vi "NoteOnNoteOff.vi"() -> ()   [LabVIEW 2015]
panel:
  in  "which cap touch sensor":i32
  in  "play note (0/1)":i32
  out "output string: play":string
  out "output string: stop playing":string
  out "index of note, initial":i32[](array[numeric])
  out "index of note":i32[](array[numeric])
  out "10-element note values":i32[](array[numeric])
  out "Interate through 36 inputs":i32
  out "10-element note values, initial":i32[](array[numeric])
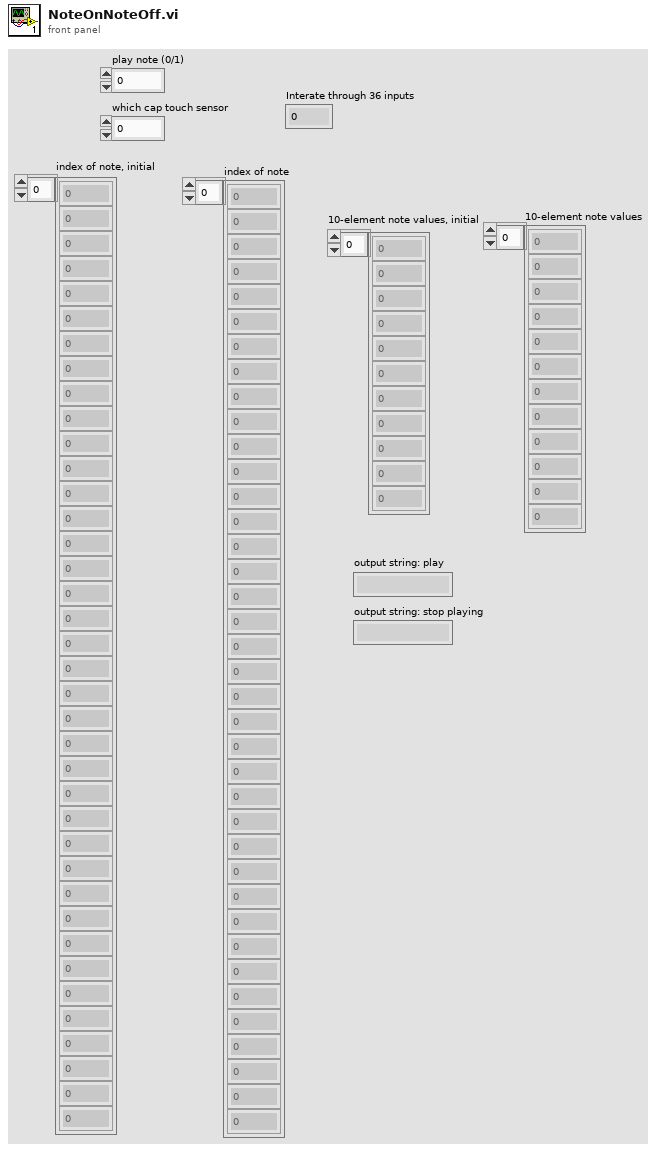
[diagram p1: front panel]
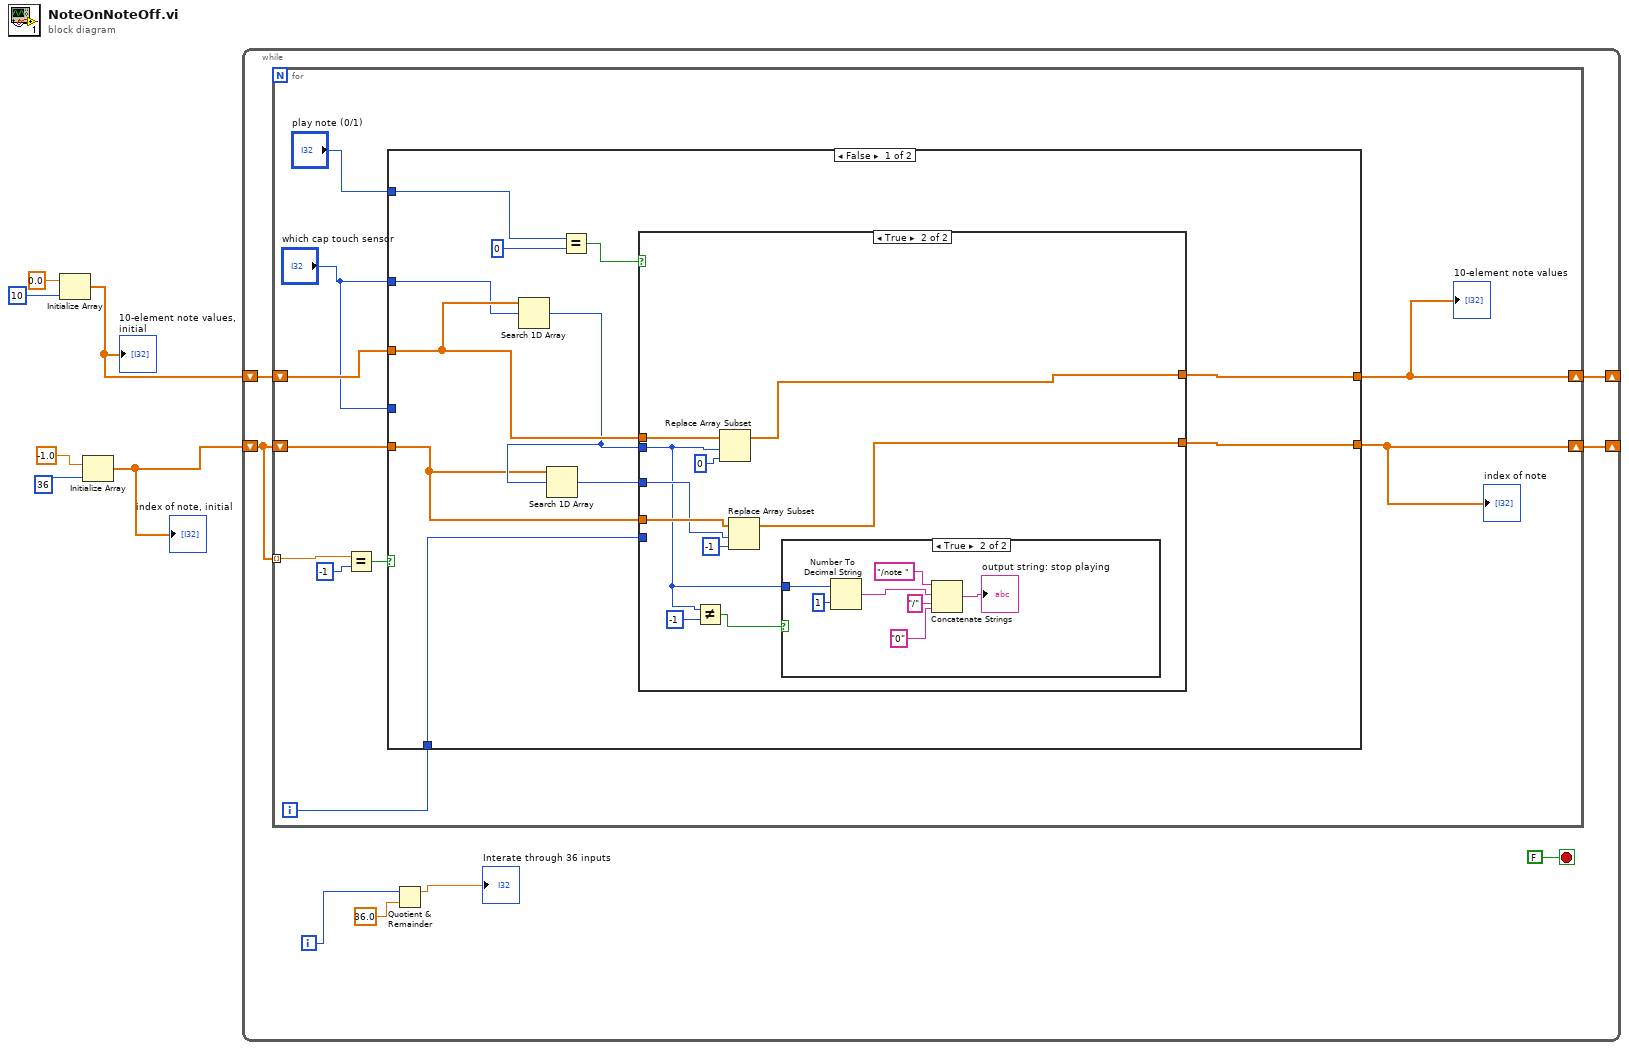
[diagram p0: block diagram]
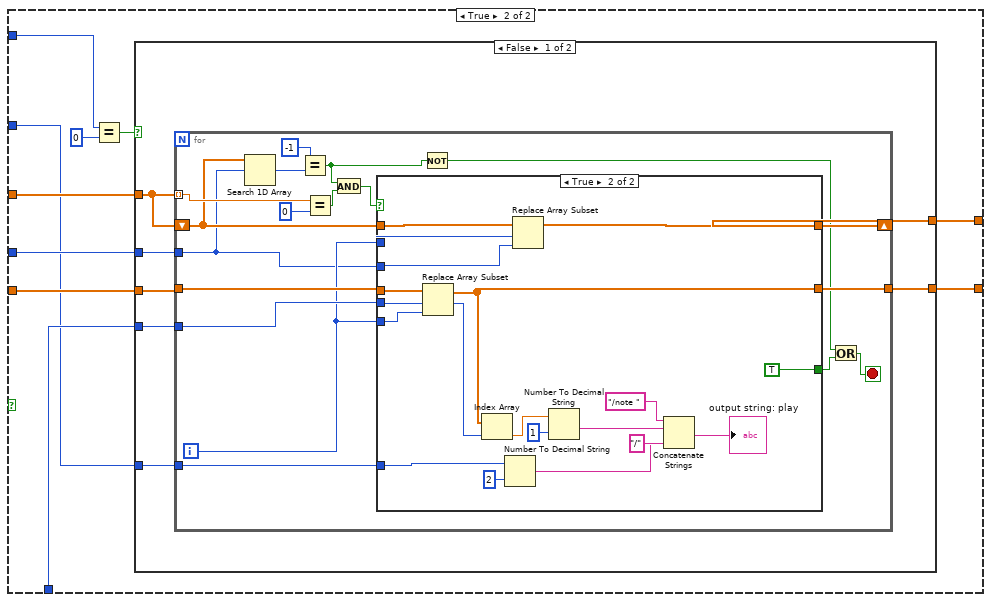
[diagram p4: hidden frame]
diagram:
  n1 = Initialize Array(0.0 ("element"), 10 ("dimension size")) -> (w1:dbl[])
  "10-element note values, initial" <- w1
  n2 = Initialize Array(-1.0 ("element"), 36 ("dimension size")) -> (w4:dbl[])
  "index of note, initial" <- w4
  n3 = while {
    shift-right: [w12] -> _
    shift-left: w1 -> [w14]
    shift-right: [w13] -> _
    shift-left: w4 -> [w10]
    i -> [w8]
    stop <- FALSE stop-if-true
    n4 = for {
      tunnel: w10 -> [w21] mode=indexing
      shift-right: [w18] -> w12
      shift-left: w14 -> [w24]
      shift-right: [w19] -> w13
      shift-left: w10 -> [w23]
      i -> [w15]
      n5 = Equal?(x=w21, y=-1) -> (x = y?=w20:bool)
      n6 = case shown="False" w20 {
        tunnel: "which cap touch sensor" -> [_ w64]
        tunnel: w24 -> [w29 w63]
        tunnel: w23 -> [w26 w62]
        tunnel: w15 -> [w34 w61]
        tunnel: "which cap touch sensor" -> [w28 w56]
        tunnel: [w32 w58] -> w18
        tunnel: [w31 w57] -> w19
        tunnel: "play note (0/1)" -> [w30 w55]
        frame False {
          n7 = Search 1D Array(1D array=w29, element=w28) -> (index of element=w27:i32)  [unwired: 1 in]
          n8 = Search 1D Array(1D array=w26, element=w27) -> (index of element=w25:i32)  [unwired: 1 in]
          n9 = Equal?(x=w30, y=0) -> (x = y?=w33:bool)
          n10 = case shown="True" w33 {
            tunnel: w29 -> [w37 w47]
            tunnel: w27 -> [_ w38]
            tunnel: w34 -> [_ _]
            tunnel: w26 -> [w36 w42]
            tunnel: [w37 w44] -> w32
            tunnel: [w36 w43] -> w31
            tunnel: w25 -> [_ w39]
            frame False {
            }
            frame True {
              n11 = Not Equal?(x=w38, y=-1) -> (x != y?=w40:bool)
              n12 = Replace Array Subset(array=w47, new element=0 ("new element/subarray"), index=w38) -> (w44:dbl[])
              n13 = Replace Array Subset(array=w42, new element=-1 ("new element/subarray"), index=w39) -> (w43:dbl[])
              n14 = case shown="True" w40 {
                tunnel: w38 -> [_ w48]
                frame False {
                }
                frame True {
                  n15 = Number To Decimal String(number=w48, width (-)=i16 1) -> (decimal integer string=w52:string)
                  n16 = Concatenate Strings("/note " ("string"), w52, "/" ("string"), "0" ("string")) -> (→"output string: stop playing":string)
                }
              }
            }
          }
        }
        frame True {
          n17 = Equal?(x=w55, y=0) -> (x = y?=w59:bool)
          n18 = case shown="False" w59 {
            tunnel: w64 -> [w71 _]
            tunnel: w63 -> [w70 w111]
            tunnel: w62 -> [w69 w110]
            tunnel: w61 -> [w68 _]
            tunnel: [w67 w111] -> w58
            tunnel: [w66 w110] -> w57
            tunnel: w56 -> [w65 _]
            frame False {
              n19 = for {
                tunnel: w70 -> [w88] mode=indexing
                tunnel: w71 -> [w80]
                tunnel: w68 -> [w86]
                shift-right: [w83] -> w67
                shift-left: w70 -> [w81]
                tunnel: w65 -> [w82]
                tunnel: w69 -> [w87]
                tunnel: [w84] -> w66
                i -> [w85]
                stop <- w74 stop-if-true
                n20 = Search 1D Array(1D array=w81, element=w80) -> (index of element=w79:i32)  [unwired: 1 in]
                n21 = Equal?(x=-1, y=w79) -> (x = y?=w73:bool)
                n22 = Equal?(x=w88, y=0) -> (x = y?=w76:bool)
                n23 = And(x=w73, y=w76) -> (x .and. y?=w77:bool)
                n24 = case shown="True" w77 {
                  tunnel: w81 -> [w91 w109]
                  tunnel: w85 -> [_ w108]
                  tunnel: w80 -> [_ w107]
                  tunnel: [_ TRUE] -> w75
                  tunnel: [w91 w105] -> w83
                  tunnel: w87 -> [w90 w98]
                  tunnel: w86 -> [_ w97]
                  tunnel: w85 -> [_ w104]
                  tunnel: [w90 w92] -> w84
                  tunnel: w82 -> [_ w96]
                  frame False {
                  }
                  frame True {
                    n25 = Replace Array Subset(array=w98, new element=w104, index=w97) -> (w92:dbl[])
                    n26 = Index Array(array=w92, index=w97) -> (element=w101:dbl)
                    n27 = Number To Decimal String(number=w96, width (-)=i16 2) -> (decimal integer string=w99:string)
                    n28 = Replace Array Subset(array=w109, new element=w107, index=w108) -> (w105:dbl[])
                    n29 = Number To Decimal String(number=w101, width (-)=i16 1) -> (decimal integer string=w100:string)
                    n30 = Concatenate Strings("/note " ("string"), w100, "/" ("string"), w99) -> (→"output string: play":string)
                  }
                }
                n31 = Not(x=w73) -> (.not. x?=w72:bool)
                n32 = Or(x=w72, y=w75) -> (x .or. y?=w74:bool)
              }
            }
            frame True {
            }
          }
        }
      }
      "10-element note values" <- w18
      "index of note" <- w19
    }
    n33 = Quotient & Remainder(x=w8, y=36.0) -> (x-y*floor(x/y)=→"Interate through 36 inputs":dbl)  [unwired: 1 out]
  }
